vi "Resideo String Data.vi"(8 "error in (no error)":errorcluster, 11 "Vesta LDO":T1) -> (0 "error out":errorcluster, 2 "Trigger Vesta Burner Control":bool, 3 "Vesta Data":string[][](array[string]))   [LabVIEW 2020]
uses:
  Type Definitions/Vesta Info.ctl
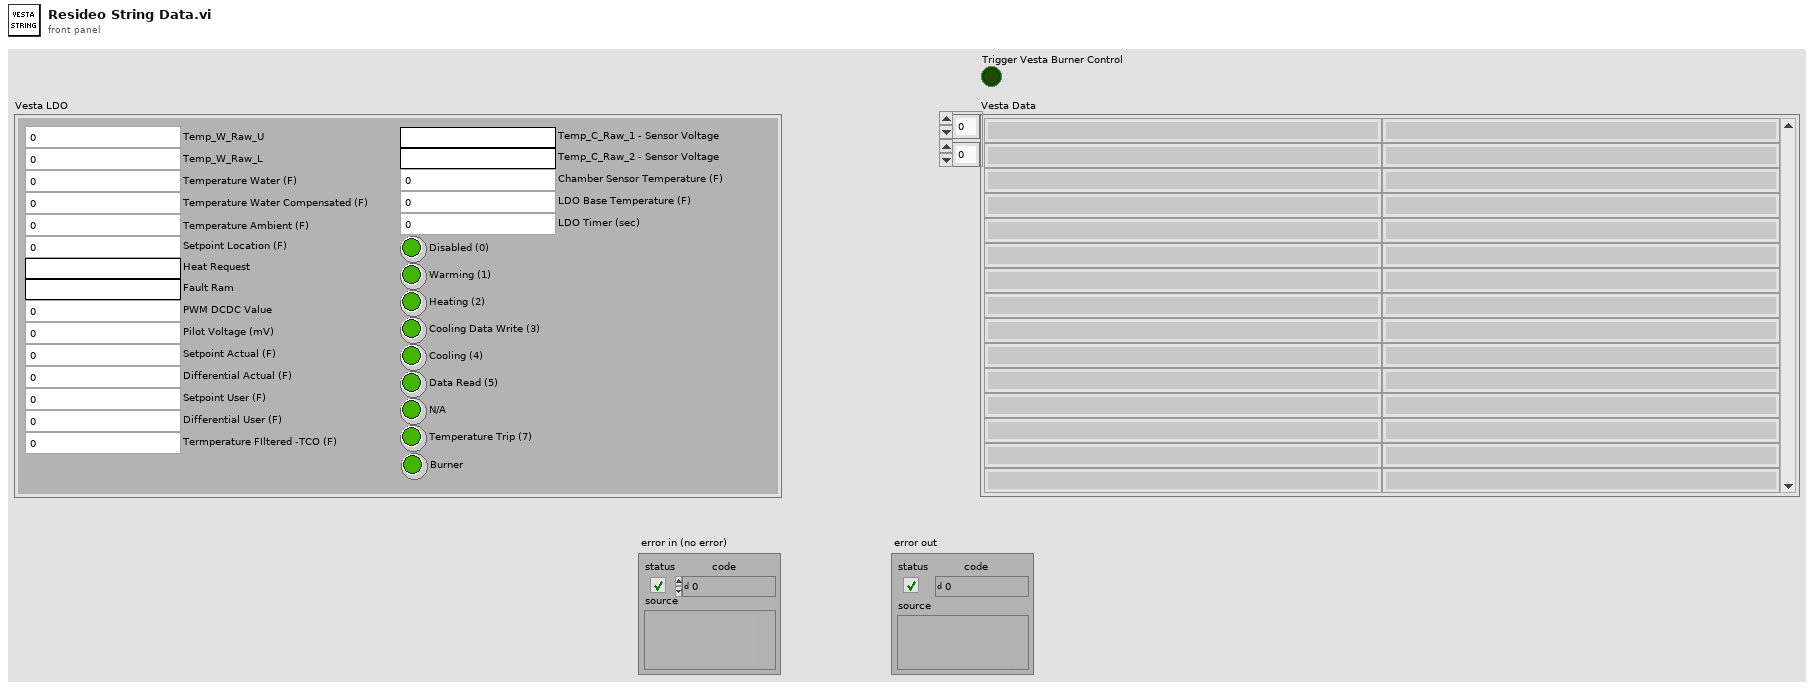
[diagram p1: front panel]
types:
  T1 = typedef "Vesta Info.ctl" = cluster{"Temp_W_Raw_U":u16, "Temp_W_Raw_L":u16, "Temperature Water (F)":dbl, "Temperature Water Compensated (F)":dbl, "Temperature Ambient (F)":dbl, "Setpoint Location (F)":dbl, "Heat Request":string, "Fault Ram":string, "PWM DCDC Value":u16, "Pilot Voltage (mV)":dbl, "Setpoint Actual (F)":dbl, "Differential Actual (F)":dbl, "Setpoint User (F)":dbl, "Differential User (F)":dbl, "Termperature FIltered -TCO (F)":dbl, "Temp_C_Raw_1 - Sensor Voltage":string, "Temp_C_Raw_2 - Sensor Voltage":string, "Chamber Sensor Temperature (F)":dbl, "LDO Base Temperature (F)":dbl, "LDO Timer (sec)":i16, "Disabled (0)":bool, "Warming (1)":bool, "Heating (2)":bool, "Cooling Data Write (3)":bool, "Cooling (4)":bool, "Data Read (5)":bool, "N/A":bool, "Temperature Trip (7)":bool, "Burner":bool}
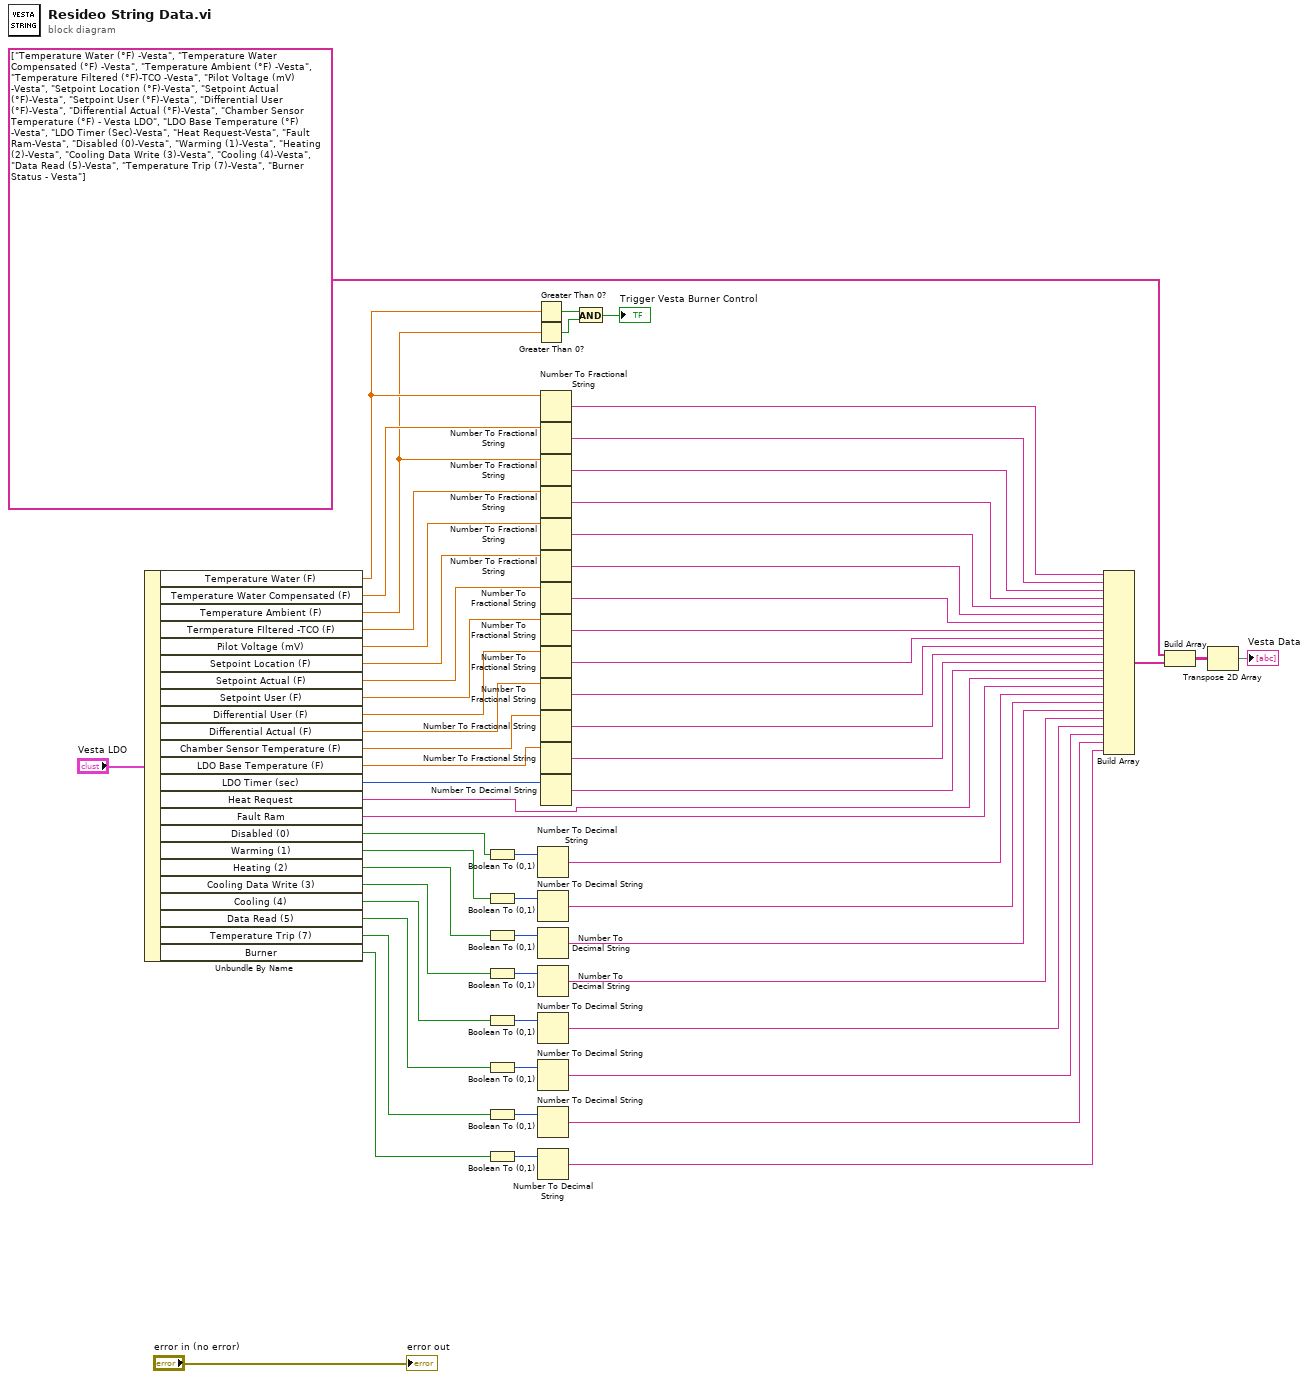
[diagram p0: block diagram]
diagram:
  n1 = Unbundle By Name("Vesta LDO") -> ("Temperature Water (F)"=w5:dbl, "Temperature Water Compensated (F)"=w59:dbl, "Temperature Ambient (F)"=w4:dbl, "Termperature FIltered -TCO (F)"=w58:dbl, "Pilot Voltage (mV)"=w57:dbl, "Setpoint Location (F)"=w56:dbl, "Setpoint Actual (F)"=w55:dbl, "Setpoint User (F)"=w54:dbl, "Differential User (F)"=w53:dbl, "Differential Actual (F)"=w52:dbl, "Chamber Sensor Temperature (F)"=w51:dbl, "LDO Base Temperature (F)"=w50:dbl, "LDO Timer (sec)"=w49:i16, "Heat Request"=w21:string, "Fault Ram"=w20:string, "Disabled (0)"=w48:bool, "Warming (1)"=w47:bool, "Heating (2)"=w46:bool, "Cooling Data Write (3)"=w45:bool, "Cooling (4)"=w44:bool, "Data Read (5)"=w43:bool, "Temperature Trip (7)"=w42:bool, "Burner"=w7:bool)
  n2 = Boolean To (0,1)(Boolean=w48) -> (0, 1=w41:i16)
  n3 = Boolean To (0,1)(Boolean=w47) -> (0, 1=w40:i16)
  n4 = Boolean To (0,1)(Boolean=w46) -> (0, 1=w39:i16)
  n5 = Boolean To (0,1)(Boolean=w45) -> (0, 1=w38:i16)
  n6 = Boolean To (0,1)(Boolean=w44) -> (0, 1=w37:i16)
  n7 = Boolean To (0,1)(Boolean=w43) -> (0, 1=w36:i16)
  n8 = Boolean To (0,1)(Boolean=w42) -> (0, 1=w35:i16)
  n9 = Boolean To (0,1)(Boolean=w7) -> (0, 1=w8:i16)
  n10 = Greater Than 0?(x=w5) -> (x > 0?=w3:bool)
  n11 = Greater Than 0?(x=w4) -> (x > 0?=w2:bool)
  n12 = Number To Decimal String(number=w41) -> (decimal integer string=w19:string)  [unwired: 1 in]
  n13 = Number To Decimal String(number=w40) -> (decimal integer string=w18:string)  [unwired: 1 in]
  n14 = Number To Decimal String(number=w39) -> (decimal integer string=w17:string)  [unwired: 1 in]
  n15 = Number To Decimal String(number=w38) -> (decimal integer string=w16:string)  [unwired: 1 in]
  n16 = Number To Decimal String(number=w37) -> (decimal integer string=w15:string)  [unwired: 1 in]
  n17 = Number To Decimal String(number=w36) -> (decimal integer string=w14:string)  [unwired: 1 in]
  n18 = Number To Decimal String(number=w35) -> (decimal integer string=w13:string)  [unwired: 1 in]
  n19 = Number To Decimal String(number=w8) -> (decimal integer string=w6:string)  [unwired: 1 in]
  n20 = Number To Fractional String(number=w5) -> (F-format string=w34:string)  [unwired: 3 in]
  n21 = Number To Fractional String(number=w59) -> (F-format string=w33:string)  [unwired: 3 in]
  n22 = Number To Fractional String(number=w4) -> (F-format string=w32:string)  [unwired: 3 in]
  n23 = Number To Fractional String(number=w58) -> (F-format string=w31:string)  [unwired: 3 in]
  n24 = Number To Fractional String(number=w57) -> (F-format string=w30:string)  [unwired: 3 in]
  n25 = Number To Fractional String(number=w56) -> (F-format string=w29:string)  [unwired: 3 in]
  n26 = Number To Fractional String(number=w55) -> (F-format string=w28:string)  [unwired: 3 in]
  n27 = Number To Fractional String(number=w54) -> (F-format string=w27:string)  [unwired: 3 in]
  n28 = Number To Fractional String(number=w53) -> (F-format string=w26:string)  [unwired: 3 in]
  n29 = Number To Fractional String(number=w52) -> (F-format string=w25:string)  [unwired: 3 in]
  n30 = Number To Fractional String(number=w51) -> (F-format string=w24:string)  [unwired: 3 in]
  n31 = Number To Fractional String(number=w50) -> (F-format string=w23:string)  [unwired: 3 in]
  n32 = Number To Decimal String(number=w49) -> (decimal integer string=w22:string)  [unwired: 1 in]
  n33 = And(x=w3, y=w2) -> (x .and. y?=→"Trigger Vesta Burner Control":bool)
  n34 = Build Array(w34, w33, w32, w31, w30, w29, w28, w27, w26, w25, w24, w23, w22, w21, w20, w19, w18, w17, w16, w15, w14, w13, w6) -> (w12:string[])
  n35 = Build Array(string[] ["Temperature Water (°F) -Vesta", "Temperature Water Compensated (°F) -Vesta", "Temperature Ambient (°F) -Vesta", "Temperature Filtered (°F)-TCO -Vesta", "Pilot Voltage (mV) -Vesta", "Setpoint Location (°F)-Vesta", "Setpoint Actual (°F)-Vesta", "Setpoint User (°F)-Vesta", "Differential User (°F)-Vesta", "Differential Actual (°F)-Vesta", "Chamber Sensor Temperature (°F) - Vesta LDO", "LDO Base Temperature (°F) -Vesta", "LDO Timer (Sec)-Vesta", "Heat Request-Vesta", "Fault Ram-Vesta", "Disabled (0)-Vesta", "Warming (1)-Vesta", "Heating (2)-Vesta", "Cooling Data Write (3)-Vesta", "Cooling (4)-Vesta", "Data Read (5)-Vesta", "Temperature Trip (7)-Vesta", "Burner Status - Vesta"], w12) -> (w10:string[][])
  n36 = Transpose 2D Array(2D array=w10) -> (transposed array=→"Vesta Data":string[][])
  "error out" <- "error in (no error)"
